vi "Turning Function.vi"   [LabVIEW 2016]
uses:
  <vilib>/NXT/Block Support/NXT_OutputPort.ctl
  <vilib>/NXT/NXTIO Xnodes/NXTIONodeSubVIs/NXTMotorRunDistance.vi
  <vilib>/NXT/Subs/LVHSConnector.ctl
  <vilib>/NXT/NXTIO Xnodes/AddressXNode/NXTIOAddress.xnode
  ENED1120.lvrbt
  <vilib>/NXT/NXTIO Xnodes/NXTIOXNode/NXTIO.xnode
  <vilib>/NXT/LegoClasses/BrickReference/BrickReference.lvclass
types:
  T1 = typedef "NXT_OutputPort.ctl" = u8
  T2 = typedef "LVHSConnector.ctl" = refnum<class "BrickReference.lvclass">
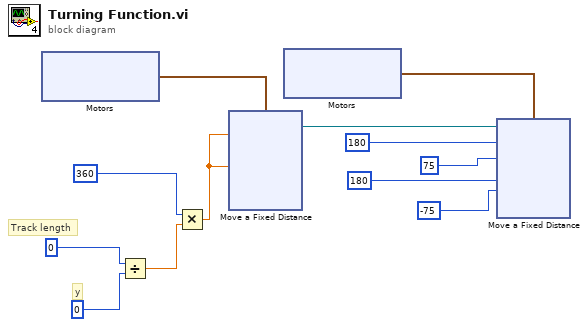
[diagram p0: block diagram]
diagram:
  # "y"
  # "Track length"
  n1 = xnode "Motors"() -> ("Motor"=w12:cluster{"Port":T1, "Port":T1})
  n2 = Divide(x=0, y=0) -> (x/y=w8:dbl)
  n3 = Multiply(x=360 ("Distance 2"), y=w8) -> (x*y=w7:dbl)
  n4 = xnode "Move a Fixed Distance"("Distance 2"=w7, "Distance 1"=w7, "Motors"=w12) -> ("NXT/EV3"=w5:T2)  [unwired: 3 in]
  n5 = xnode "Motors"() -> ("Motor"=w6:cluster{"Port":T1, "Port":T1})
  n6 = xnode "Move a Fixed Distance"("Speed 2"=i8 -75, "Speed 1"=i8 75, "Distance 2"=180, "Distance 1"=180, "Motors"=w6, "NXT/EV3"=w5) -> ()  [unwired: 1 out]
